vi "teleportRobotErForce.vi"(8 "error in (no error)":errorcluster, 10 "robot":T1, 11 "Communication in":refnum<class "Communication.lvclass">) -> (0 "error out":errorcluster, 2 "TeleportRobotArray":u8[](array[numeric]), 3 "Communication out":refnum<class "Communication.lvclass">)   [LabVIEW 2020, in "Communication.lvclass"]
uses:
  Communication.lvclass
  grSim Packet Command UDP Test Folder/grSim/grSim RobotReplacement.ctl
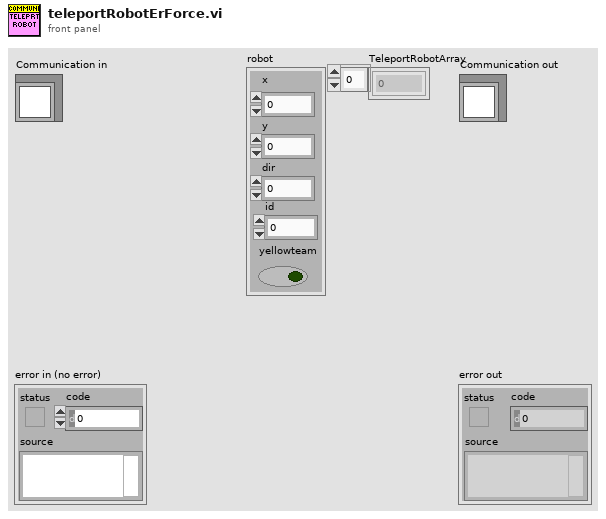
[diagram p1: front panel]
types:
  T1 = typedef "grSim RobotReplacement.ctl" = cluster{"x":dbl, "y":dbl, "dir":dbl, "yellowteam":bool, "id":u32}
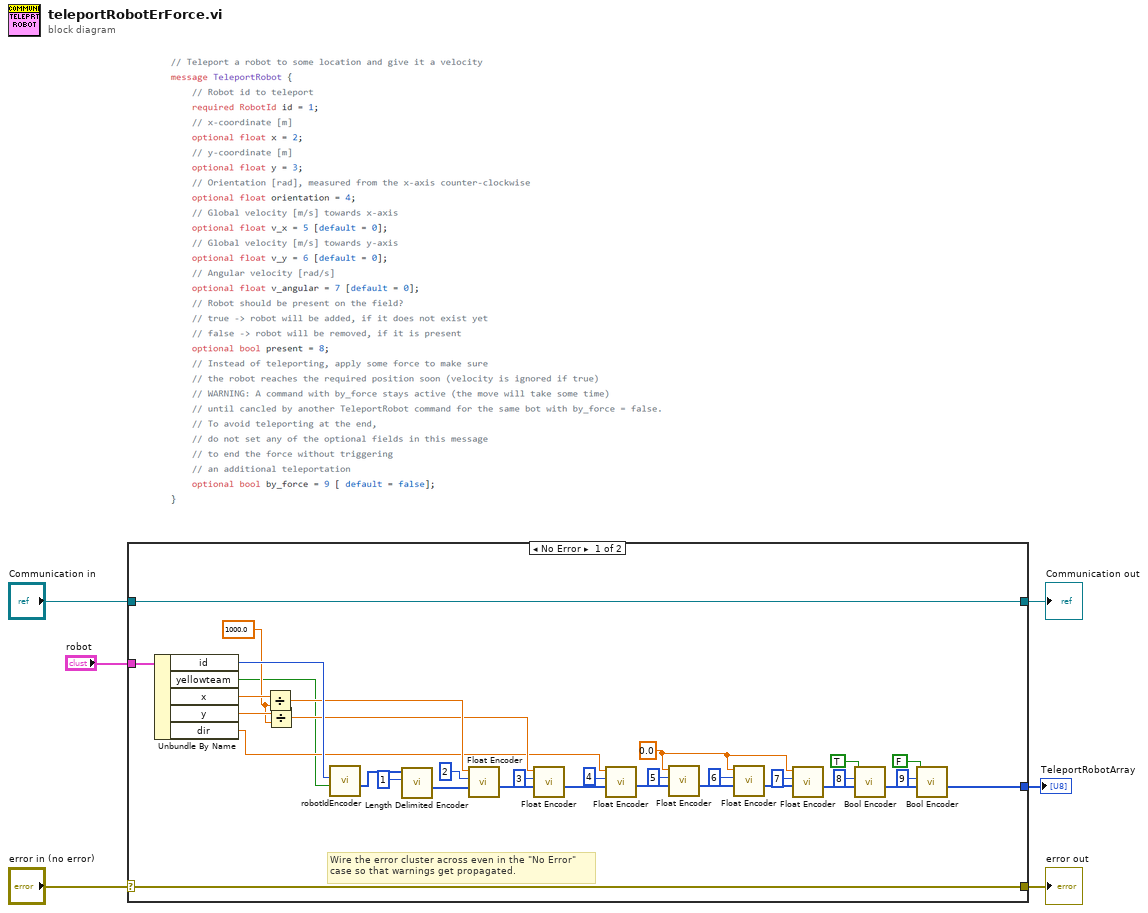
[diagram p0: block diagram]
diagram:
  n1 = case shown="No Error" "error in (no error)" {
    selector: "error in (no error)" -> [w38 w41]
    tunnel: [w38 w41] -> w5
    tunnel: [w39 w40] -> w3
    tunnel: "Communication in" -> [w39 w40]
    tunnel: "robot" -> [w37 _]
    tunnel: [w8 _] -> w1
    frame No Error {
      w16 = sgl 0.0 ("Value")
      w26 = 1000.0
      # "Wire the error cluster across even in the \"No Error\"\ncase so that warnings get propagated."
      n2 = Unbundle By Name(w37) -> ("id"=w36:u32, "yellowteam"=w7:bool, "x"=w35:dbl, "y"=w27:dbl, "dir"=w22:dbl)
      n3 = Divide(x=w35, y=w26) -> (x/y=w34:dbl)
      n4 = Divide(x=w27, y=w26) -> (x/y=w25:dbl)
      n5 = call "robotIdEncoder.vi"("yellowteam"=w7, "id"=w36) -> ("robotID Array"=w32:u8[])  [unwired: 7 in, 2 out]
      n6 = call "Length Delimited Encoder.vi"("Key"=u32 1, "Array In to be added"=w32) -> ("Array"=w31:u8[])  [unwired: 9 in]
      n7 = call "Float Encoder.vi"("Array In"=w31, "Key"=u32 2, "Value"=w34) -> ("Array"=w29:u8[])  [unwired: 8 in]
      n8 = call "Float Encoder.vi"("Array In"=w29, "Key"=u32 3, "Value"=w25) -> ("Array"=w23:u8[])  [unwired: 8 in]
      n9 = call "Float Encoder.vi"("Array In"=w23, "Key"=u32 4, "Value"=w22) -> ("Array"=w21:u8[])  [unwired: 8 in]
      n10 = call "Float Encoder.vi"("Array In"=w21, "Key"=u32 5, "Value"=w16) -> ("Array"=w19:u8[])  [unwired: 8 in]
      n11 = call "Float Encoder.vi"("Array In"=w19, "Key"=u32 6, "Value"=w16) -> ("Array"=w17:u8[])  [unwired: 8 in]
      n12 = call "Float Encoder.vi"("Array In"=w17, "Key"=u32 7, "Value"=w16) -> ("Array"=w14:u8[])  [unwired: 8 in]
      n13 = call "Bool Encoder.vi"("Array In"=w14, "Key"=u32 8, "Value"=TRUE) -> ("Array"=w11:u8[])  [unwired: 8 in]
      n14 = call "Bool Encoder.vi"("Array In"=w11, "Key"=u32 9, "Value"=FALSE) -> ("Array"=w8:u8[])  [unwired: 8 in]
    }
    frame Error {
    }
  }
  "error out" <- w5
  "Communication out" <- w3
  "TeleportRobotArray" <- w1
